vi "Connect.vi"(8 "Error In":errorcluster, 11 "object in":refnum<class "PXI-5441.lvclass">) -> (0 "Error Out":errorcluster, 3 "object out":refnum<class "PXI-5441.lvclass">)   [LabVIEW 2023, in "PXI-5441.lvlib" / "PXI-5441.lvclass"]
uses:
  PXI-5441.lvclass
  PXI-5441.lvclass/PXI-5441.ctl
  IScope_interface/IStates_interface/IStates.lvclass
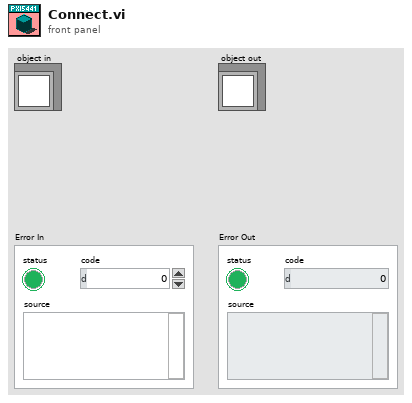
[diagram p1: front panel]
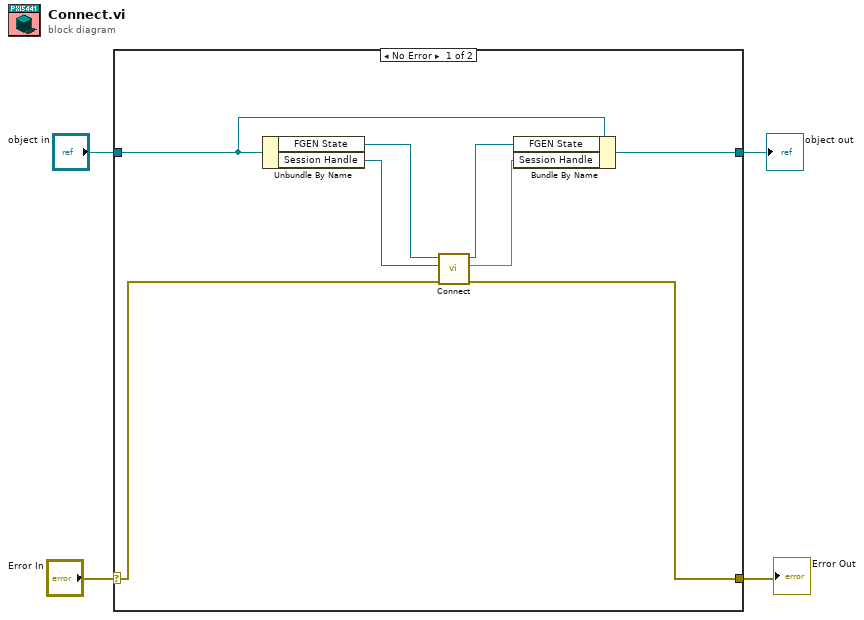
[diagram p0: block diagram]
diagram:
  n1 = case shown="No Error" "Error In" {
    selector: "Error In" -> [w12 w14]
    tunnel: [w9 w14] -> w3
    tunnel: [w10 w13] -> w1
    tunnel: "object in" -> [w11 w13]
    frame No Error {
      n2 = Unbundle By Name(w11) -> ("FGEN State"=w8:refnum<class "IStates.lvclass">, "Session Handle"=w6:refnum<k15>)
      n3 = call-dynamic "Connect.vi"("error in (no error)"=w12, 10:w6, "IStates in"=w8) -> ("error out"=w9:errorcluster, 2:w5, "IStates out"=w7:refnum<class "IStates.lvclass">)  [unwired: 6 in]
      n4 = Bundle By Name(cluster=w11, "FGEN State"=w7, "Session Handle"=w5) -> (w10:refnum<class "PXI-5441.lvclass">)
    }
    frame Error {
    }
  }
  "Error Out" <- w3
  "object out" <- w1
